vi "fgv_parameter_save-load.vi"(7 "ctl":T1(ring), 8 "error in":errorcluster, 11 "file name":string) -> (0 "error out":errorcluster, 3 "open cancelled":bool caption="취소됨")   [LabVIEW 2019]
uses:
  global_setting.vi
  <vilib>/Utility/xml.llb/Write to XML File(string).vi
  <vilib>/Utility/xml.llb/Read From XML File(string).vi
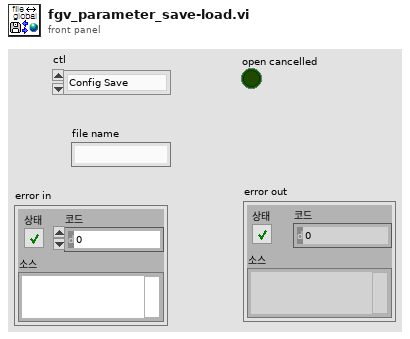
[diagram p1: front panel]
types:
  T1 = enum16{"Config Save", "Config Load", "LastRUN Save", "LastRUN Load"}
  T2 = typedef "agv_config.ctl" = cluster{"Port":refnum<visa-resource-name>, "limits":cluster{"speed limits":cluster{"max":dbl, "min":dbl}, "steer limits":cluster{"width":dbl, "offset":dbl}}, "dir":bool}
  T3 = typedef "gnss_config-2.ctl" = cluster{"Port":refnum<visa-resource-name>, "rate":u32}
  T4 = typedef "IMAQdx.ctl" = refnum<k21>
  T5 = typedef "system_hw.ctl" = cluster{"AGV":enum16{"none", "ERP42", "Scout", "SBC", "ASV"}, "Lidar 1":enum16{"none", "VLP16", "TIM571", "RPLidar A2", "RPLidar A3"}, "Lidar 2":enum16{"none", "VLP16", "TIM571", "RPLidar A2", "RPLidar A3"}, "GPS":enum16{"none", "F9P", "M8P", "PwrPak7", "19X HVS"}, "Camera":enum16{"none", "C920", "C922", "GT1290C", "MS LifeCam"}, "Joystick":enum16{"none", "joystick"}, "sound":enum16{"none", "speaker"}, "IMU":enum16{"none", "MW-AHRSv1"}, "Led":enum16{"none", "LedMatrix 8x32"}}
  T6 = typedef "joystick cfg.ctl" = cluster{"Type":enum16{"Logitech F710", "Xbox"}, "steer limit":cluster{"min":dbl, "max":dbl, "scale":dbl, "offset":dbl}, "speed limit":cluster{"min":dbl, "max":dbl, "pwm max":dbl}, "ID":i32, "joystick max":dbl}
  T7 = typedef "imu-cfg.ctl" = cluster{"Port":refnum<visa-resource-name>, "offset":dbl, "rate":u32}
  T8 = typedef "ledmatrix_data.ctl" = cluster{"ip":string, "data":string, "Port":refnum<visa-resource-name>, "time":string}
  T9 = cluster{"VLP16 cfg":cluster{"h range":cluster{i16, i16}, "v range":cluster{i8, i8}}, "TIM571 cfg":cluster{"IP":string, "h range":cluster{i16, i16}}, "AGV cfg":T2, "GPS cfg":T3, "PID cfg":cluster{"PID gains":cluster{"proportional gain (Kc)":dbl, "integral time (Ti, min)":dbl, "derivative time (Td, min)":dbl}, "PID limits":cluster{"output high":dbl, "output low":dbl}, "dt pid":u32}, "Lookahead cfg":cluster{"lookahead pts n":dbl, "lookahead distance":dbl}, "Obstacle limit range":cluster{"RL range":dbl, "Point limit":u16}, "State machine parameter":cluster{"angle adjust limit":dbl}, "waypoint group":cluster{"Waypoint array":cluster{"sel":bool, "inv":bool, "path":path}[]}, "State machine cfg":cluster{" turn angular speed":dbl, "move linear speed":dbl, "decrease factor linear speed":dbl, "adjust angle margin":dbl}, "camera cfg":cluster{"Port":T4, "Camera file":path}, "ROI-clamp":cluster{"Global Rectangle":i32[], "Contours":cluster{"Contour Type":u32, "ROI Type":u32, "Points":i32[]}[]}, "x-center":dbl, "Image Size":cluster{"x":i32, "y":i32}, "Angle deg":sgl, "Vison cfg":cluster{"Clamp Settings":cluster{"Contrast":i32, "Filter width":i32, "Steepness":i32, "Subsampling Ratio":u32, "Show Search Area":bool, "Show Search Lines":bool, "Show Edges Found":bool, "Show Result":bool}, "Range":cluster{"Lower value":sgl, "Upper value":sgl}, "N of Erosion 1":i32, "N of Erosion 2":i32}, "RPLidar cfg":cluster{"port":refnum<visa-resource-name>, "dt":u32, "update":u8, "speed":u16, "rate ":u32}, "HW info":T5, "Joystick cfg":T6, "IMU cfg":T7, "ledmatrix cfg":T8}
  T10 = enum16{"open", "replace", "create", "open or create", "replace or create", "replace or create with confirmation"}
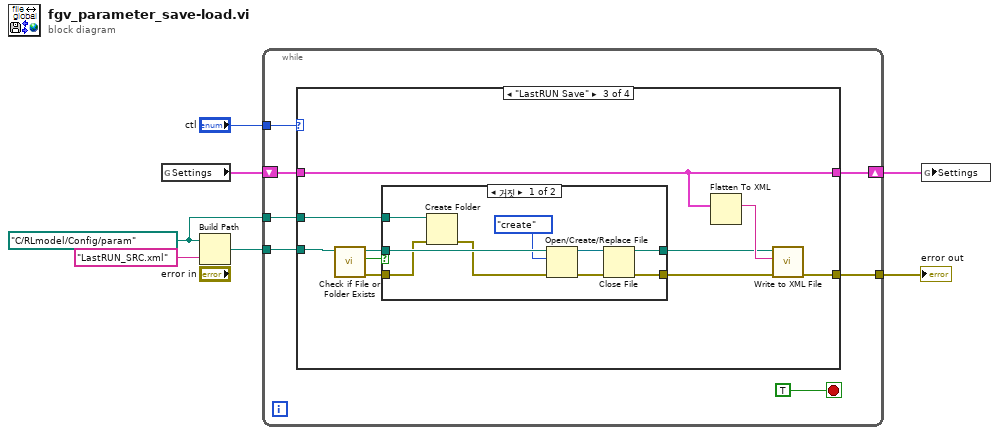
[diagram p0: block diagram]
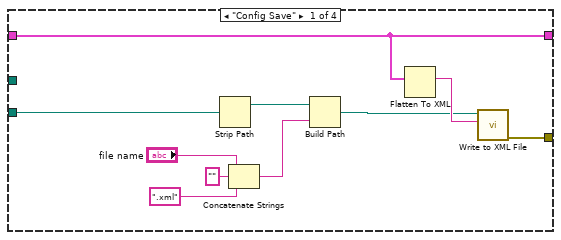
[diagram p2: hidden frame]
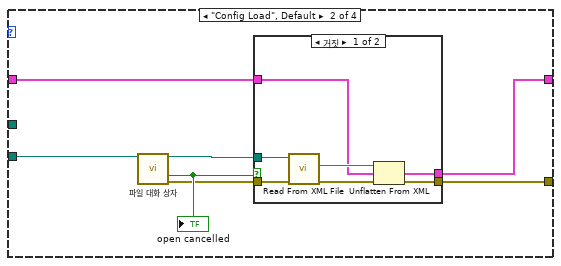
[diagram p3: hidden frame]
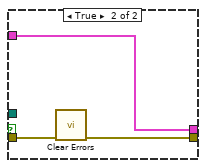
[diagram p4: hidden frame]
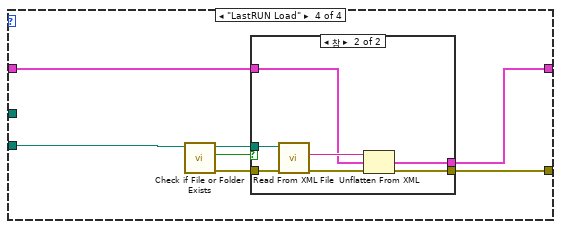
[diagram p6: hidden frame]
diagram:
  w1 = path "C:/RLmodel/Config/param" ("XML File Path")
  n1 = global read "global_setting.vi" "Settings"() -> (w3:T9)
  n2 = Build Path(base path=w1, name or relative path="LastRUN_SRC.xml" ("이름 또는 상대 경로")) -> (appended path=w4:path)
  n3 = while {
    tunnel: [w14] -> w7
    tunnel: "ctl" -> [w13]
    tunnel: w4 -> [w11]
    shift-right: [w10] -> w2
    shift-left: w3 -> [w12]
    tunnel: w1 -> [w8]
    stop <- TRUE stop-if-true
    n4 = case shown="\"LastRUN Save\"" w13 {
      tunnel: w12 -> [w19 w28 w45 w69]
      tunnel: w11 -> [w22 w31 w44 w63]
      tunnel: [w23 w26 w46 w67] -> w14
      tunnel: [w19 w25 w45 w68] -> w10
      tunnel: w8 -> [_ _ w42 _]
      frame "Config Save" {
        n5 = Strip Path(path=w22) -> (stripped path=w21:path)  [unwired: 1 out]
        n6 = Concatenate Strings("file name", "" ("문자열"), ".xml" ("문자열")) -> (w20:string)
        n7 = Build Path(base path=w21, name or relative path=w20) -> (appended path=w16:path)
        n8 = Flatten To XML(anything=w19) -> (xml string=w24:string)
        n9 = call-poly <vilib>:"Write to XML File.vi"("XML Input"=w24, "XML File Path"=w16) -> ("error out"=w23:errorcluster)  [unwired: 7 in, 2 out]
      }
      frame "Config Load", Default {
        n10 = call "파일 대화 상자"("start path"=w31) -> ("selected path"=w29:path, "cancelled"=w30:bool, "error out"=w27:errorcluster)  [unwired: 11 in, 1 out]
        "open cancelled" <- w30
        n11 = case shown="거짓" w30 {
          tunnel: w29 -> [w37 _]
          tunnel: w28 -> [w36 w41]
          tunnel: [w35 w41] -> w25
          tunnel: w27 -> [w33 w40]
          tunnel: [w32 w39] -> w26
          frame False {
            n12 = call-poly <vilib>:"Read From XML File.vi"("error in (no error)"=w33, "XML File Path"=w37) -> ("error out"=w34:errorcluster, "XML Elements"=w38:string)  [unwired: 7 in, 1 out]
            n13 = Unflatten From XML(xml string=w38, type=w36, error in (no error)=w34) -> (value=w35:T9, error out=w32:errorcluster)
          }
          frame True {
            n14 = call <vilib>:"Clear Errors.vi"("error in (no error)"=w40) -> ("error out"=w39:errorcluster)  [unwired: 5 in, 1 out]
          }
        }
      }
      frame "LastRUN Save" {
        n15 = call <vilib>:"Check if File or Folder Exists.vi"("path"=w44) -> ("error out"=w50:errorcluster, "file or folder exists?"=w48:bool, "dup path"=w49:path)  [unwired: 8 in]
        n16 = case shown="거짓" w48 {
          tunnel: w50 -> [w53 w62]
          tunnel: w49 -> [w60 w61]
          tunnel: [w55 w62] -> w47
          tunnel: [w56 w61] -> w43
          tunnel: w42 -> [w54 _]
          frame False {
            n17 = Create Folder(path (use dialog)=w54, error in=w53) -> (error out=w52:errorcluster)  [unwired: 1 in, 2 out]
            n18 = Open/Create/Replace File(file path (use dialog)=w60, error in=w52, operation (0:open)=T10."create" ("동작(0:open)")) -> (refnum out=w57:refnum<file>, error out=w58:errorcluster)  [unwired: 3 in, 1 out]
            n19 = Close File(refnum=w57, error in=w58) -> (path=w56:path, error out=w55:errorcluster)
          }
          frame True {
          }
        }
        n20 = Flatten To XML(anything=w45) -> (xml string=w51:string)
        n21 = call-poly <vilib>:"Write to XML File.vi"("error in (no error)"=w47, "XML Input"=w51, "XML File Path"=w43) -> ("error out"=w46:errorcluster)  [unwired: 6 in, 2 out]
      }
      frame "LastRUN Load" {
        n22 = call <vilib>:"Check if File or Folder Exists.vi"("path"=w63) -> ("error out"=w64:errorcluster, "file or folder exists?"=w65:bool, "dup path"=w66:path)  [unwired: 8 in]
        n23 = case shown="참" w65 {
          tunnel: w69 -> [_ w76]
          tunnel: [_ w75] -> w68
          tunnel: [w70 w73] -> w67
          tunnel: w66 -> [_ w72]
          tunnel: w64 -> [w70 w71]
          frame False {
          }
          frame True {
            n24 = call-poly <vilib>:"Read From XML File.vi"("error in (no error)"=w71, "XML File Path"=w72) -> ("error out"=w74:errorcluster, "XML Elements"=w77:string)  [unwired: 7 in, 1 out]
            n25 = Unflatten From XML(xml string=w77, type=w76, error in (no error)=w74) -> (value=w75:T9, error out=w73:errorcluster)
          }
        }
      }
    }
  }
  "error out" <- w7
  n26 = global write "global_setting.vi" "Settings"(w2) -> ()
